vi "Gradient Read Array.vi"(8 "error in":errorcluster, 11 "Temperature Gradient in":refnum<class "Temperature Gradient.lvclass">) -> (0 "error out":errorcluster, 1 "Changed or First Call?":bool, 2 "Temperature SP":dbl[](array[numeric]), 3 "Temperature Gradient out":refnum<class "Temperature Gradient.lvclass">)   [LabVIEW 2023, in "Temperature Gradient.lvclass"]
uses:
  Temperature Gradient.lvclass
  Temperature Gradient.lvclass/Temperature Gradient.ctl
  Parents/Gradient/Gradient.lvclass
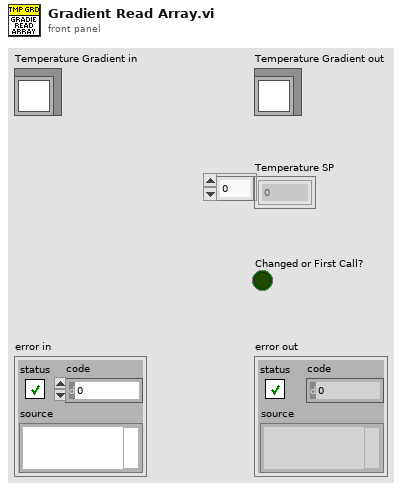
[diagram p1: front panel]
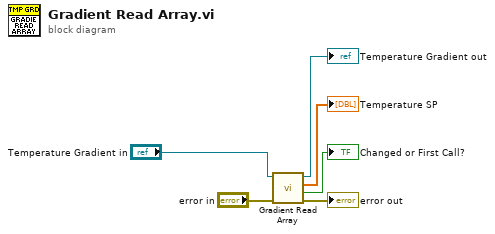
[diagram p0: block diagram]
diagram:
  n1 = call-parent "Gradient Read Array.vi"("error in"="error in", "Gradient in"="Temperature Gradient in") -> ("error out"=→"error out":errorcluster, "Changed or First Call?"=→"Changed or First Call?":bool, "Current SP"=→"Temperature SP":dbl[], "Gradient out"=→"Temperature Gradient out":refnum<class "Temperature Gradient.lvclass">)  [unwired: 6 in]
